vi "Sentry.vi"() -> ()   [LabVIEW 2020]
panel:
  in  "Path":path
  out "Numeric":dbl
  in  "Audio File Path":string
  in  "module path 2":path
  out "Boolean":bool
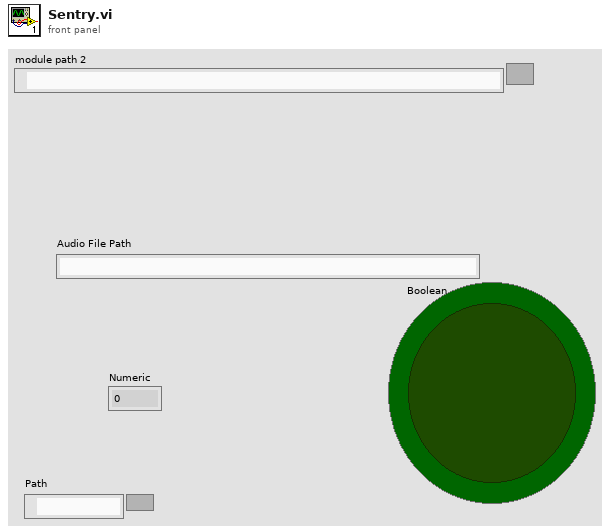
[diagram p1: front panel]
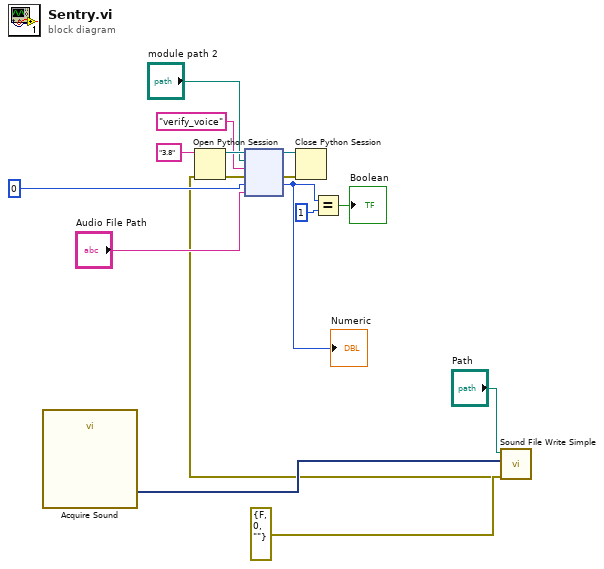
[diagram p0: block diagram]
diagram:
  n1 = call "Acquire Sound"() -> ("Data"=w4:dynamicdata)  [unwired: 18 in, 1 out]
  n2 = call <vilib>:"Sound File Write Simple.vi"("error in (no error)"=errorcluster {"status"=FALSE, "code"=0, "source"=""}, "data"=w4, "path"="Path") -> ("error out"=w1:errorcluster)  [unwired: 7 in, 1 out]
  n3 = Open Python Session(python version="3.8" ("Python version"), 3:w1) -> (session out=w15:refnum<k35>, error out=w5:errorcluster)  [unwired: 1 in]
  n4 = node(w15, "module path 2", "verify_voice" ("function name"), w5, 0, "Audio File Path") -> (w14:refnum<k35>, w7:errorcluster, w6:i32)  [unwired: 1 in, 2 out]
  "Numeric" <- w6
  n5 = Close Python Session(session in=w14, error in=w7) -> ()  [unwired: 1 out]
  n6 = Equal?(x=w6, y=1) -> (x = y?=→"Boolean":bool)
